vi "LHWE Latent Heat of Water Evaporation (KJ to Kg).vi"(1 "Tceg":dbl[unit]) -> (0 "LHWE":dbl[unit])   [LabVIEW 2018]
panel:
  out "TC-W 3":dbl[unit]=647.3
  out "LHWE\nLatent Heat of Water Evaporation;\nLHWE=2501*((TCW-Tk)/(TCW-273.15))**0.38":dbl[unit](knob)
  out "Temprature Of Input Air\nKelvin Degree":dbl[unit](slide) scale=273.0..373.0
  out "Tk":dbl[unit]
  out "Temprature Of Input Air\nCentigrade Degree":dbl[unit](slide) scale=0.0..100.0
  out "TC-W 2":dbl[unit]=647.3
  out "TC-W":dbl[unit]=647.3
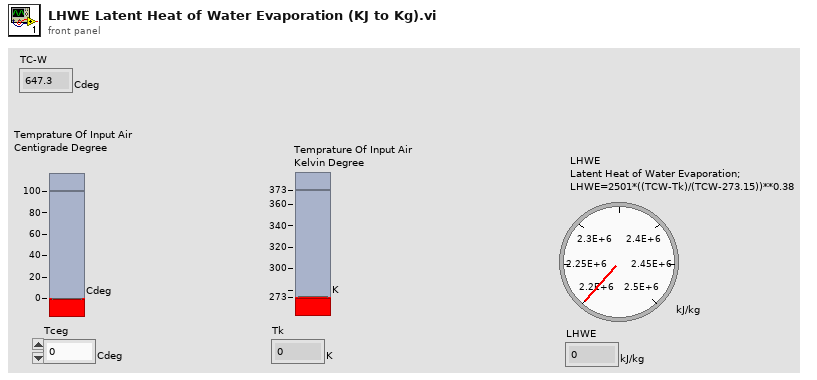
[diagram p1: front panel]
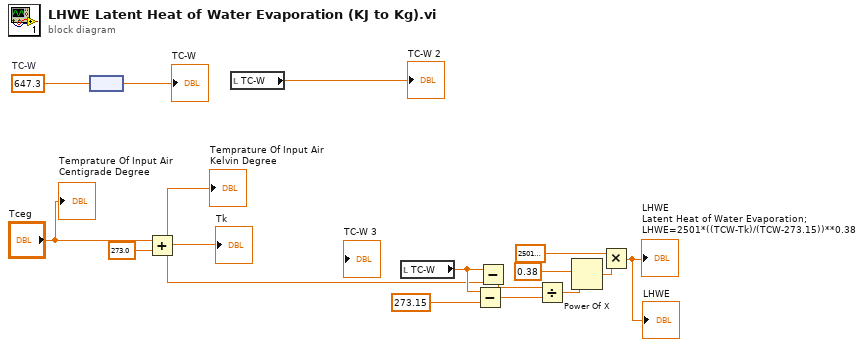
[diagram p0: block diagram]
diagram:
  w15 = 647.3  # TC-W
  n1 = node(w15) -> (→"TC-W":dbl[unit])
  n2 = Add(x="Tceg", y=dbl[unit] 273.0) -> (x+y=w2:dbl[unit])
  "Tk" <- w2
  "Temprature Of Input Air\nKelvin Degree" <- w2
  n3 = local read "TC-W"() -> (→"TC-W 2":dbl[unit])
  n4 = local read "TC-W"() -> (w8:dbl[unit])
  n5 = Subtract(x=w8, y=dbl[unit] 273.15) -> (x-y=w9:dbl[unit])
  n6 = Subtract(x=w8, y=w2) -> (x-y=w10:dbl[unit])
  n7 = Divide(x=w10, y=w9) -> (x/y=w4:dbl)
  n8 = Power Of X(1:w4, 2:0.38 ("y")) -> (0:w6:dbl)
  n9 = Multiply(x=dbl[unit] 2501000.0, y=w6) -> (x*y=→"LHWE\nLatent Heat of Water Evaporation;\nLHWE=2501*((TCW-Tk)/(TCW-273.15))**0.38" →"LHWE":dbl[unit])
  "Temprature Of Input Air\nCentigrade Degree" <- "Tceg"
